vi "FindChessboardCornersGreyscale.vi"(5 "Flags (Default - Adaptive Threshold, Normalize and Fast Check)":T3[](array[typedef])=[enum."CALIB_CB_ADAPTIVE_THRESH", enum."CALIB_CB_NORMALIZE_IMAGE", enum."CALIB_CB_FAST_CHECK"], 7 "Chessboard Corners Info":T2, 8 "error in (no error)":errorcluster, 11 "Greyscale Image in":T4) -> (0 "error out":errorcluster, 2 "Points":T1[](array[typedef]), 3 "Greyscale Image":T4)   [LabVIEW 2020, in "feature_detection.lvlib"]
doc: "Detect the Chessboard in the Image and return the <b>Internal</b> Corner Points."
uses:
  feature_detection.lvlib
  image/Greyscale Image.ctl
  Find Chessboard Corners Flags.ctl
  Chessboard Corner Info.ctl
  common/Image Point (Float).ctl
  ca99938f-1423-42fb-b653-ffd1f73e2bb5.vi
  <vilib>/Utility/error.llb/Error Cluster From Error Code.vi
  common/common.lvlib
  image/image.lvlib
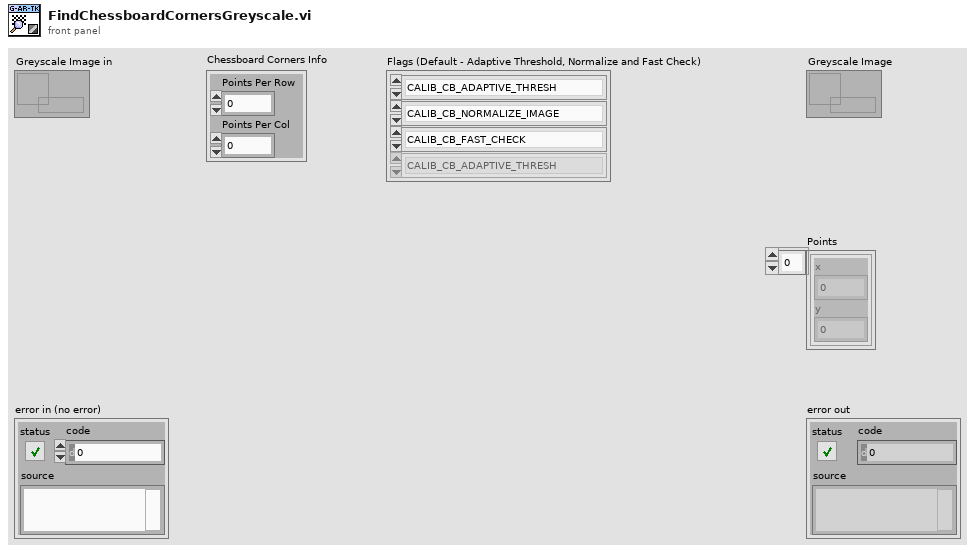
[diagram p1: front panel]
types:
  T1 = typedef "common.lvlib/Image Point (Float).ctl" = cluster{"x":dbl, "y":dbl}
  T2 = typedef "feature_detection.lvlib/Chessboard Corner Info.ctl" = cluster{"Points Per Row":u8, "Points Per Col":u8}
  T3 = typedef "feature_detection.lvlib/Find Chessboard Corners Flags.ctl" = enum8{"CALIB_CB_ADAPTIVE_THRESH", "CALIB_CB_NORMALIZE_IMAGE", "CALIB_CB_FILTER_QUADS", "CALIB_CB_FAST_CHECK"}
  T4 = typedef "image.lvlib/Greyscale Image.ctl" = refnum<data-value>
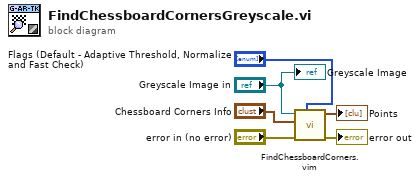
[diagram p0: block diagram]
diagram:
  n1 = call "FindChessboardCorners.vim"("Flags (Default - Adaptive Threshold, Normalize and Fast Check)"="Flags (Default - Adaptive Threshold, Normalize and Fast Check)", "error in (no error)"="error in (no error)", "Chessboard Corners Info"="Chessboard Corners Info", "Src"="Greyscale Image in") -> ("error out"=→"error out":errorcluster, "Points"=→"Points":T1[])  [unwired: 6 in]
  "Greyscale Image" <- "Greyscale Image in"
